vi "Actuate.vi"(0 "Actuator in":refnum<class "Actuator.lvclass">, 5 "FC1 ILC in":refnum<class "ILC.lvclass">, 7 "FC2 ILC in":refnum<class "ILC.lvclass">, 9 "Actuate Arguments":T3 {"FC2 Measured Value" format="%.3f"; "Lateral Demand" format="%.3f"; "FC1 Measured Value" format="%.3f"; "Axial Demand" format="%.3f"}, 11 "error in (no error)":errorcluster) -> (4 "Actuator out":refnum<class "Actuator.lvclass">, 6 "FC1 ILC out":refnum<class "ILC.lvclass">, 8 "FC2 ILC out":refnum<class "ILC.lvclass">, 10 "Actuate Results":T1 {"FC2 Demand" format="%.3f"; "FC1 Demand" format="%.3f"}, 15 "error out":errorcluster)   [LabVIEW 2015, in "Actuator.lvclass"]
uses:
  Actuator.lvclass
  <userlib>/Common/ILC/ILC/ILC.lvclass
  Typedefs/Actuate Arguments.ctl
  Typedefs/Actuate Results.ctl
  Typedefs/Cylinder Results.ctl
  Typedefs/FAMT Typedefs.lvlib
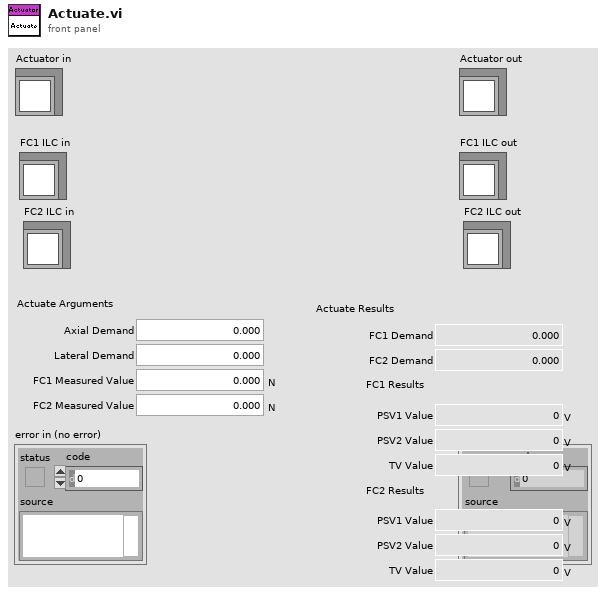
[diagram p1: front panel]
types:
  T1 = typedef "FAMT Typedefs.lvlib/Actuate Results.ctl" = cluster{"FC1 Demand":dbl, "FC2 Demand":dbl, "FC1 Results":T2, "FC2 Results":T2}
  T2 = typedef "FAMT Typedefs.lvlib/Cylinder Results.ctl" = cluster{"PSV1 Value":dbl[unit], "PSV2 Value":dbl[unit], "TV Value":dbl[unit]}
  T3 = typedef "FAMT Typedefs.lvlib/Actuate Arguments.ctl" = cluster{"Axial Demand":dbl, "Lateral Demand":dbl, "FC1 Measured Value":dbl[unit], "FC2 Measured Value":dbl[unit]}
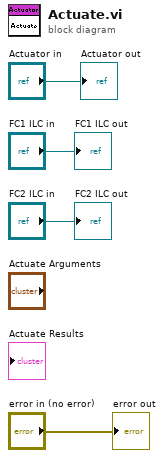
[diagram p0: block diagram]
diagram:
  "error out" <- "error in (no error)"
  "Actuator out" <- "Actuator in"
  "FC1 ILC out" <- "FC1 ILC in"
  "FC2 ILC out" <- "FC2 ILC in"
